vi "Add Digital Pattern.vi"(8 "error in (no error)":errorcluster, 10 "Page Data in":T1 {"Node Ptr" format="%.0x"}, 11 "State queue in":string[](array[string])) -> (0 "error out":errorcluster, 2 "Page Data out":T1 {"Node Ptr" format="%.0x"}, 3 "State queue out":string[](array[string]))   [LabVIEW 2019, in "Engine Simulation Toolkit System Explorer.lvlib"]
uses:
  Engine Simulation Toolkit System Explorer.lvlib
  Digital Patterns Page Data.ctl
  <vilib>/NI VeriStand/Custom Device API/Custom Device Item Ref.ctl
  Digital Pattern.ctl
  Digital Pattern Base.ctl
  Digital Pattern Remove Edge.ctl
  Digital Pattern Add Pulse.ctl
  <vilib>/NI VeriStand/Custom Device API/Custom Device Channel Type.ctl
  Shared/Constants and GUIDs.vi
  Shared/Properties.vi
  <vilib>/NI VeriStand/Custom Device API/Set Item Property (String).vi
  <vilib>/NI VeriStand/Custom Device API/Custom Device API.lvlib
  Shared/Engine Simulation Toolkit Shared.lvlib
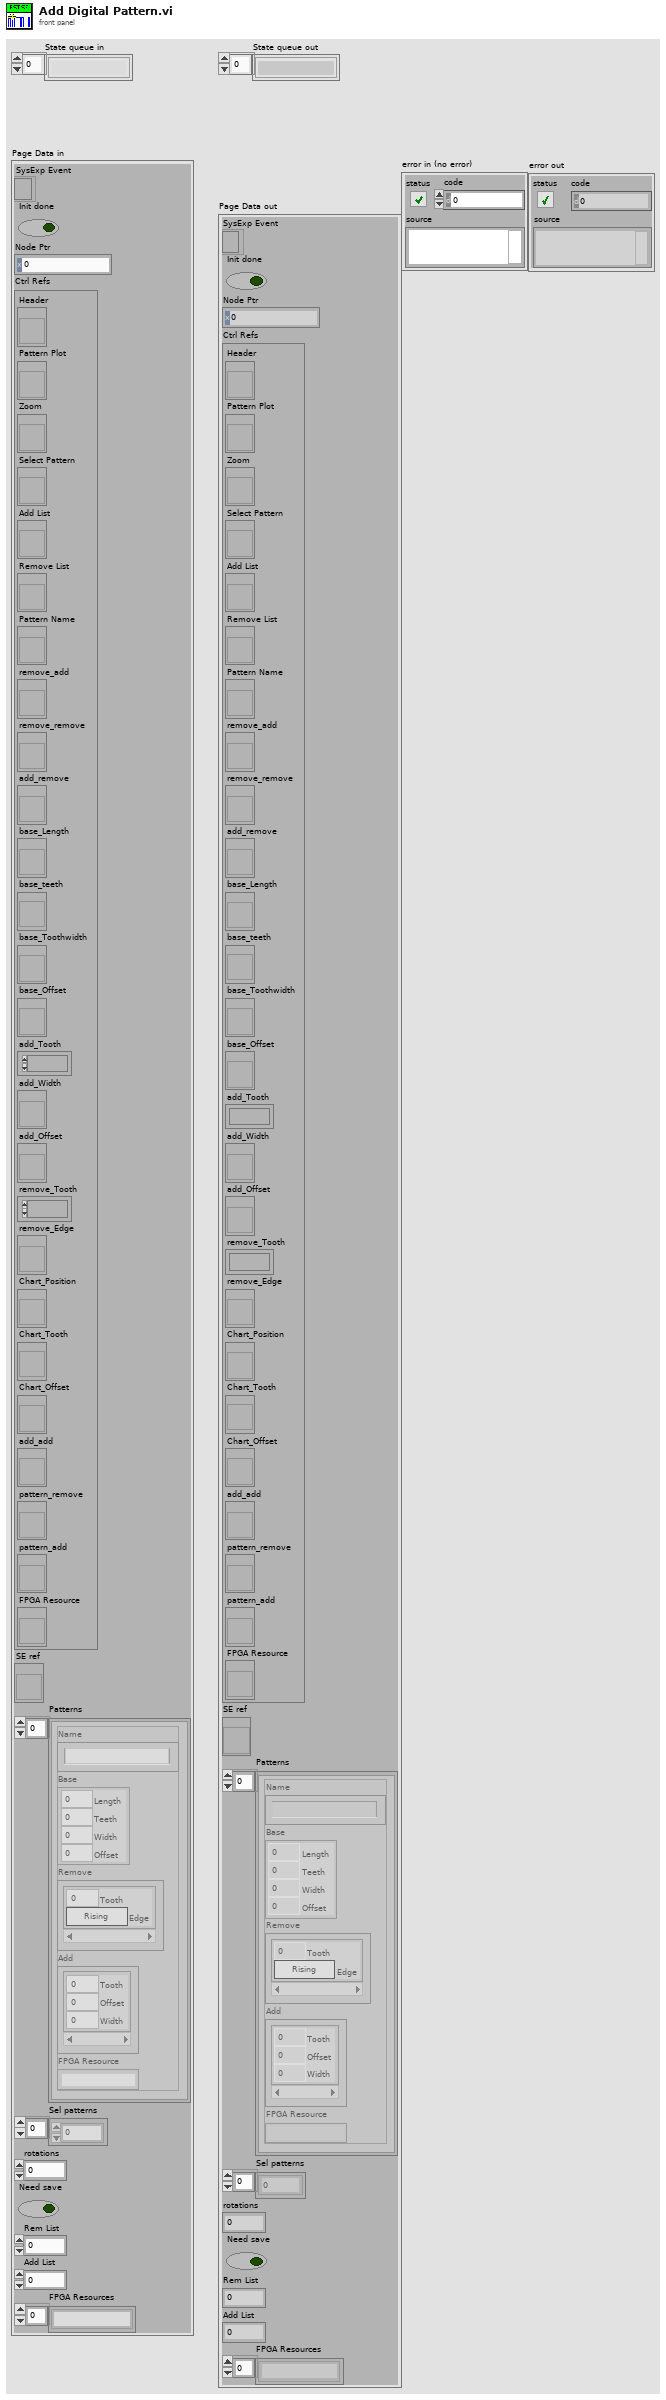
[diagram p1: front panel]
types:
  T1 = typedef "Engine Simulation Toolkit System Explorer.lvlib/Digital Patterns Page Data.ctl" = cluster{"SysExp Event":refnum<event-registration>, "Init done":bool, "Node Ptr":T2, "Ctrl Refs":cluster{"Header":refnum<vi>, "Pattern Plot":refnum<vi>, "Zoom":refnum<vi>, "Select Pattern":refnum<vi>, "Add List":refnum<vi>, "Remove List":refnum<vi>, "Pattern Name":refnum<vi>, "remove_add":refnum<vi>, "remove_remove":refnum<vi>, "add_remove":refnum<vi>, "base_Length":refnum<vi>, "base_teeth":refnum<vi>, "base_Toothwidth":refnum<vi>, "base_Offset":refnum<vi>, "add_Tooth":refnum<vi>, "add_Width":refnum<vi>, "add_Offset":refnum<vi>, "remove_Tooth":refnum<vi>, "remove_Edge":refnum<vi>, "Chart_Position":refnum<vi>, "Chart_Tooth":refnum<vi>, "Chart_Offset":refnum<vi>, "add_add":refnum<vi>, "pattern_remove":refnum<vi>, "pattern_add":refnum<vi>, "FPGA Resource":refnum<vi>}, "SE ref":refnum<vi>, "Patterns":T3[], "Sel patterns":i32[], "rotations":u16, "Need save":bool, "Rem List":i32, "Add List":i32, "FPGA Resources":string[]}
  T2 = typedef "Custom Device API.lvlib/Custom Device Item Ref.ctl" = u64
  T3 = typedef "Engine Simulation Toolkit System Explorer.lvlib/Digital Pattern.ctl" = cluster{"Name":string, "Base":T4, "Remove":T5[], "Add":T6[], "FPGA Resource":string}
  T4 = typedef "Engine Simulation Toolkit System Explorer.lvlib/Digital Pattern Base.ctl" = cluster{"Length":dbl, "Teeth":u16, "Width":dbl, "Offset":dbl}
  T5 = typedef "Engine Simulation Toolkit System Explorer.lvlib/Digital Pattern Remove Edge.ctl" = cluster{"Tooth":u16, "Edge":bool}
  T6 = typedef "Engine Simulation Toolkit System Explorer.lvlib/Digital Pattern Add Pulse.ctl" = cluster{"Tooth":u16, "Offset":dbl, "Width":dbl}
  T7 = typedef "Custom Device API.lvlib/Custom Device Channel Type.ctl" = enum16{"Input", "Output"}
  T8 = typedef "Engine Simulation Toolkit Shared.lvlib/Bitfile EST Version.ctl" = enum16{"1.0", "1.1", "1.2", "1.3", "1.4"}
  T9 = typedef "Engine Simulation Toolkit Shared.lvlib/Channel.ctl" = cluster{"Name":string, "Units":string, "Default":dbl, "Description":string, "Scalable":bool}
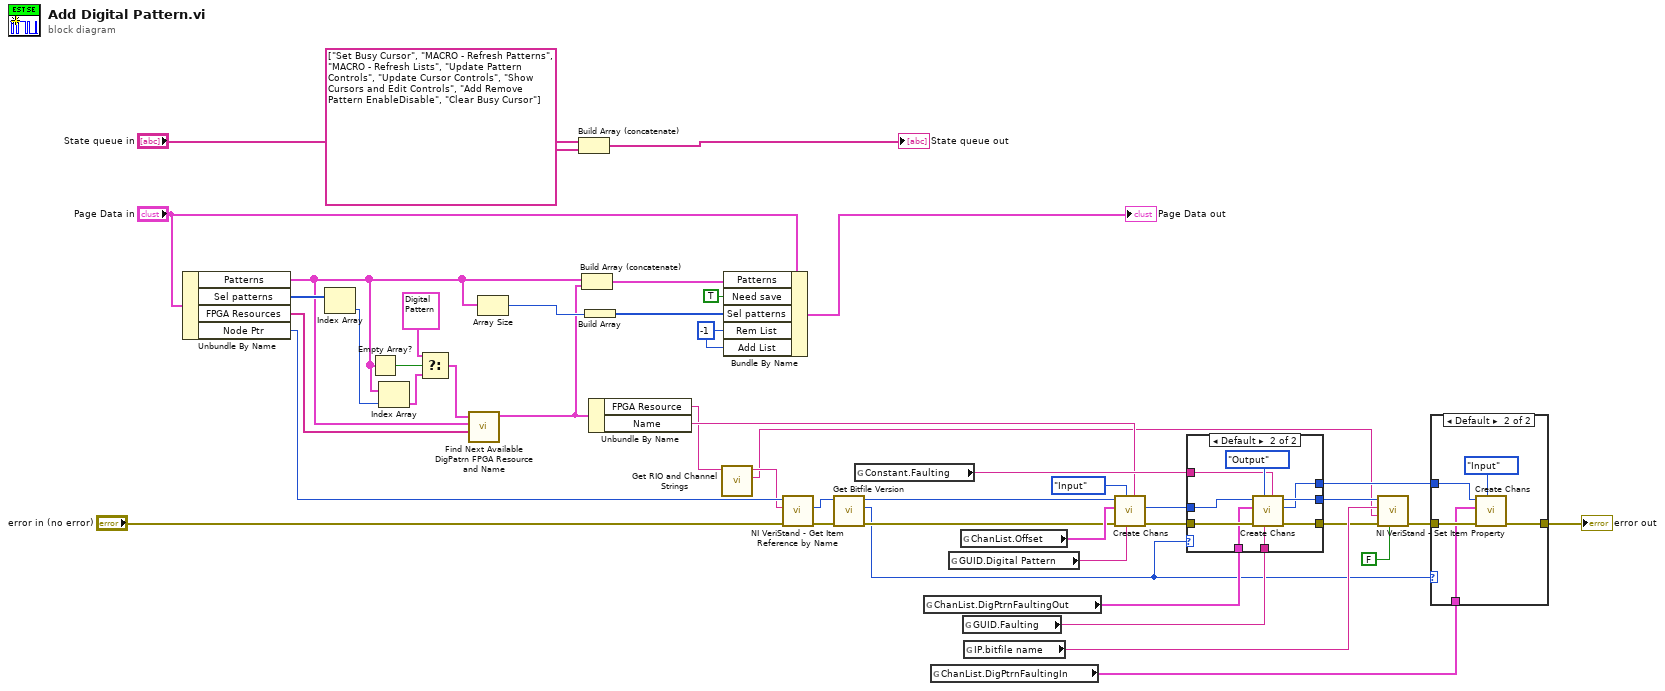
[diagram p0: block diagram]
diagram:
  w45 = -1 ("Rem List")
  n1 = Unbundle By Name("Page Data in") -> ("Patterns"=w31:T3[], "Sel patterns"=w40:i32[], "FPGA Resources"=w32:string[], "Node Ptr"=w5:T2)
  n2 = Index Array(array=w40) -> (element=w42:i32)  [unwired: 1 in]
  n3 = Empty Array?(array=w31) -> (empty?=w29:bool)
  n4 = Index Array(array=w31, index=w42) -> (element=w39:T3)
  n5 = Select(t=T3 {"Name"="New Pattern", "Base"={"Length"=360.0, "Teeth"=60, "Width"=1.0, "Offset"=-0.5}, "Remove"=[{"Tooth"=58, "Edge"=FALSE}, {"Tooth"=59, "Edge"=FALSE}], "Add"=[], "FPGA Resource"=""} ("s? t:f"), s=w29, f=w39) -> (s? t:f=w30:T3)
  n6 = call "Find Next Available DigPatrn FPGA Resource and Name.vi"("FPGA Resources"=w32, "Patterns"=w31, "New Pattern in"=w30) -> ("New Pattern out"=w28:T3)  [unwired: 8 in]
  n7 = Array Size(array=w31) -> (size(s)=w46:i32)
  n8 = Build Array (concatenate)("State queue in", string[] ["Set Busy Cursor", "MACRO - Refresh Patterns", "MACRO - Refresh Lists", "Update Pattern Controls", "Update Cursor Controls", "Show Cursors and Edit Controls", "Add Remove Pattern EnableDisable", "Clear Busy Cursor"]) -> (→"State queue out":string[])
  n9 = Build Array (concatenate)(w31, w28) -> (w41:T3[])
  n10 = Build Array(w46) -> (w43:i32[])
  n11 = Unbundle By Name(w28) -> ("FPGA Resource"=w2:string, "Name"=w3:string)
  n12 = call "Get RIO and Channel Strings.vi"("rio/channel"=w2) -> ("channel"=w1:string, "rio"=w4:string)  [unwired: 9 in]
  n13 = Bundle By Name(cluster="Page Data in", "Patterns"=w41, "Need save"=TRUE, "Sel patterns"=w43, "Rem List"=w45, "Add List"=w45) -> (→"Page Data out":T1)
  n14 = call <vilib>:"NI VeriStand - Get Item Reference by Name.vi"("error in (no error)"="error in (no error)", "Item Name"=w4, "Parent Ref in"=w5) -> ("error out"=w8:errorcluster, "Item Ref"=w7:T2)  [unwired: 5 in, 2 out]
  n15 = call "Get Bitfile Version.vi"("error in (no error)"=w8, "Item Ref in"=w7) -> ("error out"=w12:errorcluster, "EST version enum"=w10:T8, "Item Ref out"=w11:T2)  [unwired: 6 in, 1 out]
  n16 = global read "Constants and GUIDs.vi" "Constant.Faulting"() -> (w9:string)
  n17 = global read "Constants and GUIDs.vi" "ChanList.DigPtrnFaultingOut"() -> (w18:T9[])
  n18 = global read "Constants and GUIDs.vi" "ChanList.DigPtrnFaultingIn"() -> (w15:T9[])
  n19 = global read "Constants and GUIDs.vi" "GUID.Digital Pattern"() -> (w25:string)
  n20 = global read "Constants and GUIDs.vi" "ChanList.Offset"() -> (w26:T9[])
  n21 = global read "Constants and GUIDs.vi" "GUID.Faulting"() -> (w13:string)
  n22 = global read "Properties.vi" "IP.bitfile name"() -> (w23:string)
  n23 = call "Create Chans.vi"("New Section Name (none)"=w3, "new section GUID (\"\":del prot)"=w25, "Type"=Custom_Device_Channel_Type."Input", "error in (no error)"=w12, "Channels"=w26, "Section Ptr"=w11) -> ("error out"=w24:errorcluster, "new section ref"=w20:T2)  [unwired: 2 in, 2 out]
  n24 = case shown="Default" w10 {
    tunnel: w24 -> [w47 w57]
    tunnel: [w47 w56] -> w21
    tunnel: w20 -> [w48 w55]
    tunnel: [w48 w54] -> w19
    tunnel: w18 -> [_ w53]
    tunnel: [_ w51] -> w16
    tunnel: w13 -> [_ w50]
    tunnel: w9 -> [_ w49]
    frame "1.0".."1.2" {
    }
    frame Default {
      n25 = call "Create Chans.vi"("New Section Name (none)"=w49, "new section GUID (\"\":del prot)"=w50, "Type"=Custom_Device_Channel_Type."Output", "error in (no error)"=w57, "Channels"=w53, "Section Ptr"=w55) -> ("error out"=w56:errorcluster, "new section ref"=w51:T2, "Section Ptr dup"=w54:T2)  [unwired: 2 in, 1 out]
    }
  }
  n26 = call-poly <vilib>:"NI VeriStand - Set Item Property.vi"("Binary String (T)"=FALSE, "error in (no error)"=w21, "Value"=w1, "Property Name"=w23, "Item Ref in"=w19) -> ("error out"=w17:errorcluster)  [unwired: 4 in, 2 out]
  n27 = case shown="Default" w10 {
    tunnel: w17 -> [w58 w63]
    tunnel: w16 -> [_ w62]
    tunnel: w15 -> [_ w61]
    tunnel: [w58 w59] -> w14
    frame "1.0".."1.2" {
    }
    frame Default {
      n28 = call "Create Chans.vi"("Type"=Custom_Device_Channel_Type."Input", "error in (no error)"=w63, "Channels"=w61, "Section Ptr"=w62) -> ("error out"=w59:errorcluster)  [unwired: 4 in, 3 out]
    }
  }
  "error out" <- w14
